vi "HowToAdjustAngle.vi"(10 "Desired Sailing Regime":T1, 11 "Current Sailing Regime":T1) -> (3 "Desired Sailing Regime 2":T1)   [LabVIEW 2013]
doc: "This VI looks at the regime that the boat is in and the desired regime, then determines how best to get there from the current position.\n\nFor example, if we are on a port tack and want to be on a starboard tack, this VI should tell the boat to tack to port. If the boat needs to go from starboard tack to close to running with the wind over the starboard bow, this VI should tell the boat to go into the 'Turn w/o crossing wind' behavior, to port.\n\nEric Schneider, Feb. 2014"
uses:
  Data/TypeDefs/Sailing Regimes.ctl
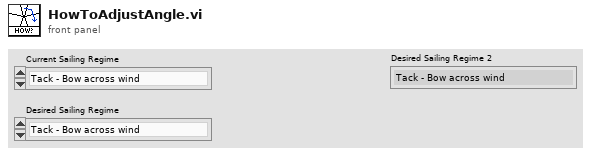
[diagram p1: front panel]
types:
  T1 = typedef "Sailing Regimes.ctl" = enum16{"Tack - Bow across wind", "Upwind - Port Tack", "Turn between Upwind/Reach - Port Tack", "Reach - Port Tack", "Turn between Reach/Run - Port Tack", "Run - Port Tack", "Jibe - Stern across wind", "Run - Starboard Tack", "Turn between Reach/Run - Starboard Tack", "Reach - Starboard Tack", "Turn between Upwind/Reach - Starboard Tack", "Upwind - Starboard Tack"}
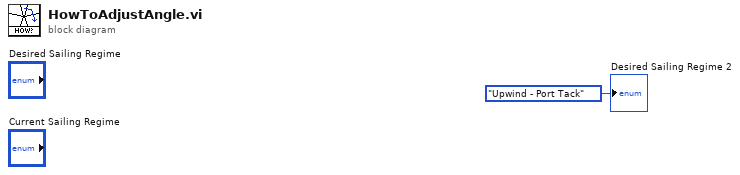
[diagram p0: block diagram]
diagram:
  "Desired Sailing Regime 2" <- Sailing_Regimes."Upwind - Port Tack" ("Desired Sailing Regime 2")
